vi "Read Y_A.vi"(11 "reg in":refnum<class "bronkhorst_reg_2.lvclass">) -> (2 "Y_A":dbl step=1.0, 3 "reg out":refnum<class "bronkhorst_reg_2.lvclass">)   [LabVIEW 2019, in "control.lvlib" / "bronkhorst_reg_2.lvclass"]
uses:
  bronkhorst_reg_2.lvclass
  bronkhorst_reg_2.lvclass/bronkhorst_reg_2.ctl
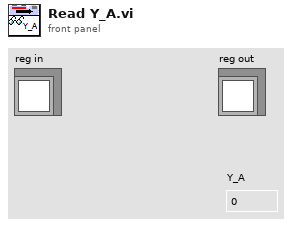
[diagram p1: front panel]
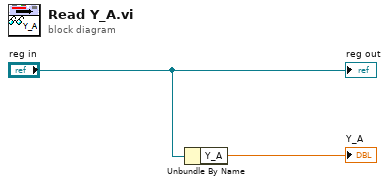
[diagram p0: block diagram]
diagram:
  n1 = Unbundle By Name("reg in") -> ("Y_A"=→"Y_A":dbl)
  "reg out" <- "reg in"
